vi "SpeedFinder.vi"(2 "Angle(degrees)":dbl, 3 "Vision Distance(in)":dbl) -> (0 "error out":errorcluster, 1 "Initial Speed(in/s)":dbl)   [LabVIEW 2015]
doc: "Returns the speed required to score a high goal for a given launch angle, or an error if the angle is not high enough to score."
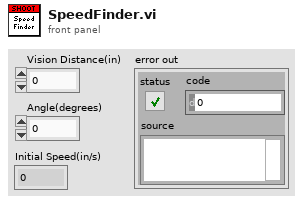
[diagram p1: front panel]
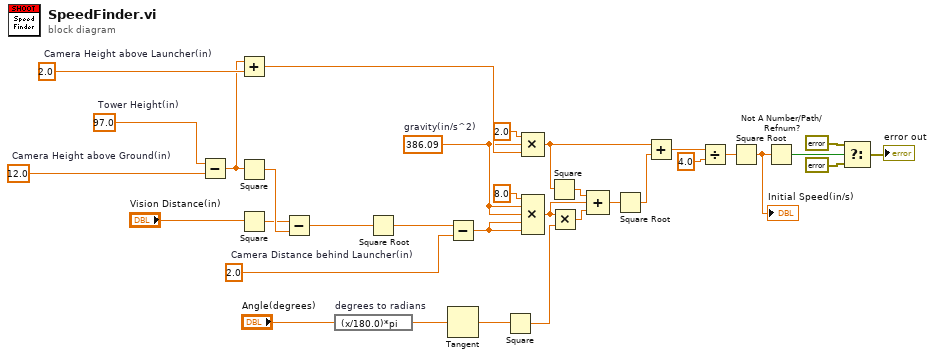
[diagram p0: block diagram]
diagram:
  w21 = 2.0  # Camera Height above Launcher(in)
  w10 = 386.09  # gravity(in/s^2)
  w33 = 2.0  # Camera Distance behind Launcher(in)
  w31 = 12.0  # Camera Height above Ground(in)
  w32 = 97.0  # Tower Height(in)
  n1 = Subtract(x=w32, y=w31) -> (x-y=w20:dbl)
  n2 = Add(x=w20, y=w21) -> (x+y=w15:dbl)
  n3 = Square(x=w20) -> (x^2=w28:dbl)
  n4 = Square(x="Vision Distance(in)") -> (x^2=w27:dbl)
  n5 = Subtract(x=w27, y=w28) -> (x-y=w29:dbl)
  n6 = expression code="(x/180.0)*pi" "degrees to radians"("Angle(degrees)") -> (w3:dbl)
  n7 = Square Root(x=w29) -> (sqrt(x)=w26:dbl)
  n8 = Subtract(x=w26, y=w33) -> (x-y=w9:dbl)
  n9 = Tangent(1:w3) -> (0:w6:dbl)
  n10 = Square(x=w6) -> (x^2=w5:dbl)
  n11 = Compound Arithmetic op=MULTIPLY(2.0 ("value"), w10, w15) -> (w12:dbl)
  n12 = Compound Arithmetic op=MULTIPLY(8.0 ("value"), w10, w10, w9, w9) -> (w7:dbl)
  n13 = Square(x=w12) -> (x^2=w13:dbl)
  n14 = Multiply(x=w7, y=w5) -> (x*y=w8:dbl)
  n15 = Compound Arithmetic op=ADD(w13, w7, w8) -> (w2:dbl)
  n16 = Square Root(x=w2) -> (sqrt(x)=w14:dbl)
  n17 = Add(x=w12, y=w14) -> (x+y=w17:dbl)
  n18 = Divide(x=w17, y=4.0) -> (x/y=w18:dbl)
  n19 = Square Root(x=w18) -> (sqrt(x)=w1:dbl)
  "Initial Speed(in/s)" <- w1
  n20 = Not A Number/Path/Refnum?(number/path/refnum=w1) -> (NaN/Path/Refnum?=w25:bool)
  n21 = Select(t=errorcluster {"status"=TRUE, "code"=9001, "source"="Unable to score!"} ("error constant"), s=w25, f=errorcluster {"status"=FALSE, "code"=0, "source"=""}) -> (s? t:f=→"error out":errorcluster)
